vi "LightController.vi"() -> ()   [LabVIEW 2018]
uses:
  Content/TypeDef/EventTypeDef.ctl
  HASS-LV-WS_integration.lvlib
  <vilib>/MediaMongrels Ltd/WebSockets/WebSockets/WebSockets.lvlib
panel:
  in  "Pulse":bool
  out "Light State":T1
  in  "Color Temperature":u16(slide) scale=153.0..500.0
  in  "Brightness":u8(slide) scale=0.0..255.0
  in  "Light Entity ID":string
  in  "Light Control":bool
  out "Event Data":string
  out "Event Name":string
  in  "Stop Button":bool
  out "Connection Authenticated?":bool
  out "Connection Result":string
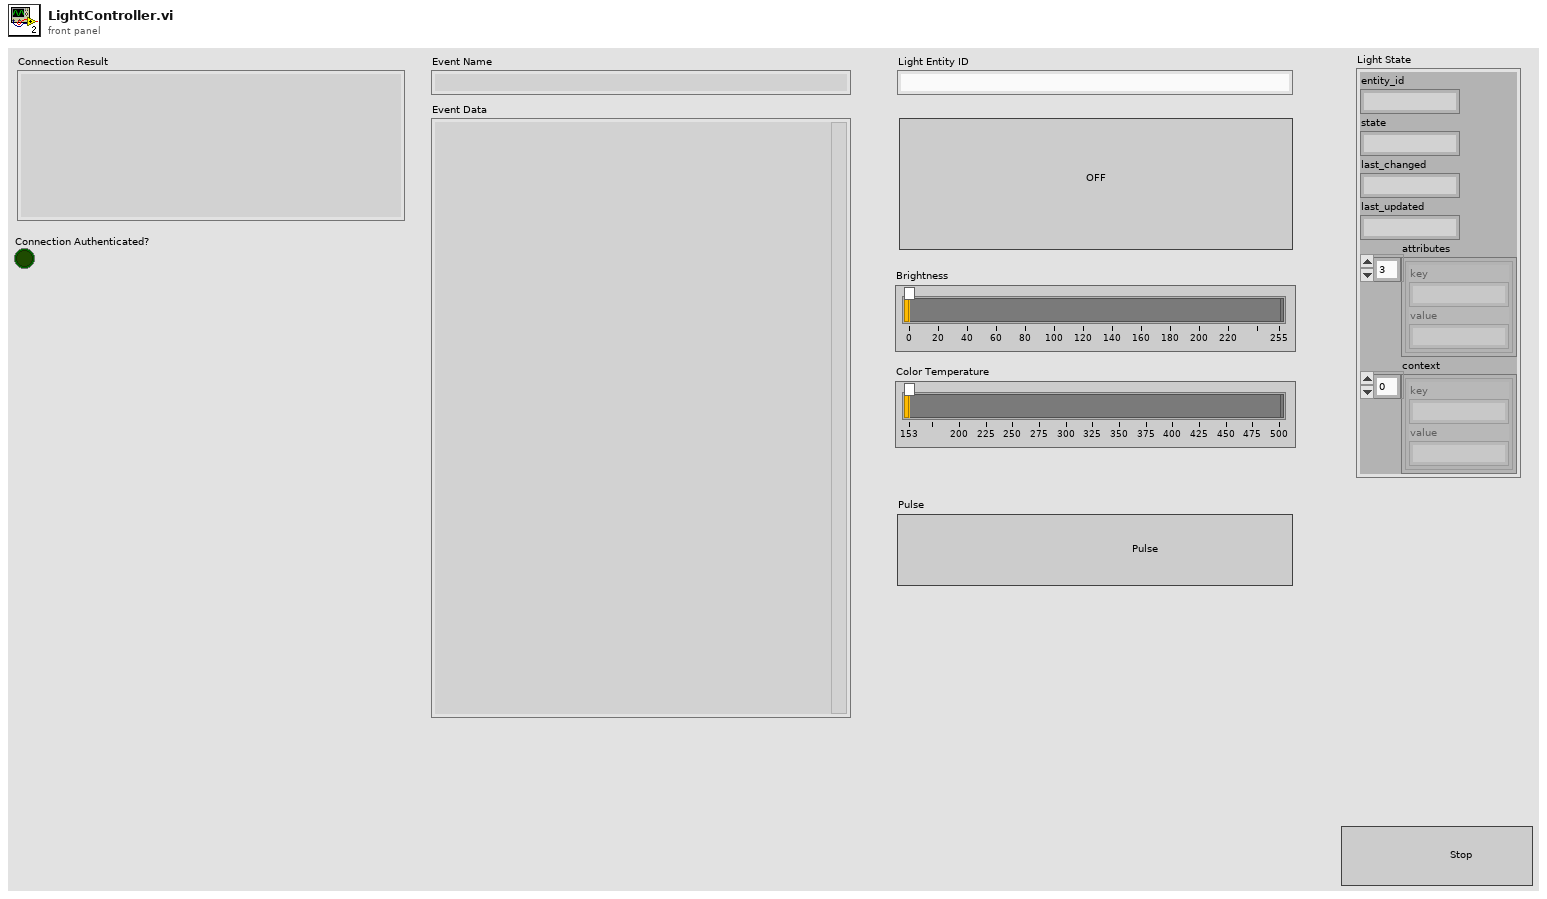
[diagram p1: front panel]
types:
  T1 = cluster{"entity_id":string, "state":string, "last_changed":string, "last_updated":string, "attributes":cluster{"key":string, "value":string}[], "context":cluster{"key":string, "value":string}[]}
  T2 = typedef "HASS-LV-WS_integration.lvlib/ReferencesTypeDef.ctl" = cluster{"user event":refnum<user-event>, "send queue":refnum<queue>, "receive queue":refnum<queue>, "TCP Network Connection":refnum<k5>, "ws engine notifier ":refnum<notifier>, "Event Registration Refnum":refnum<event-registration>}
  T3 = typedef "HASS-LV-WS_integration.lvlib/EventTypeDef.ctl" = cluster{"Data":variant, "Command":string}
  T4 = cluster{"Service Domain":string, "Service":string, "Optional - Service Data (JSON string)":string}
  T5 = cluster{"entity_id":string, "state":string, "last_changed":string, "last_updated":string, "attributes":cluster{"key":string, "value":string}[], "context":cluster{"key":string, "value":string}[]}[]
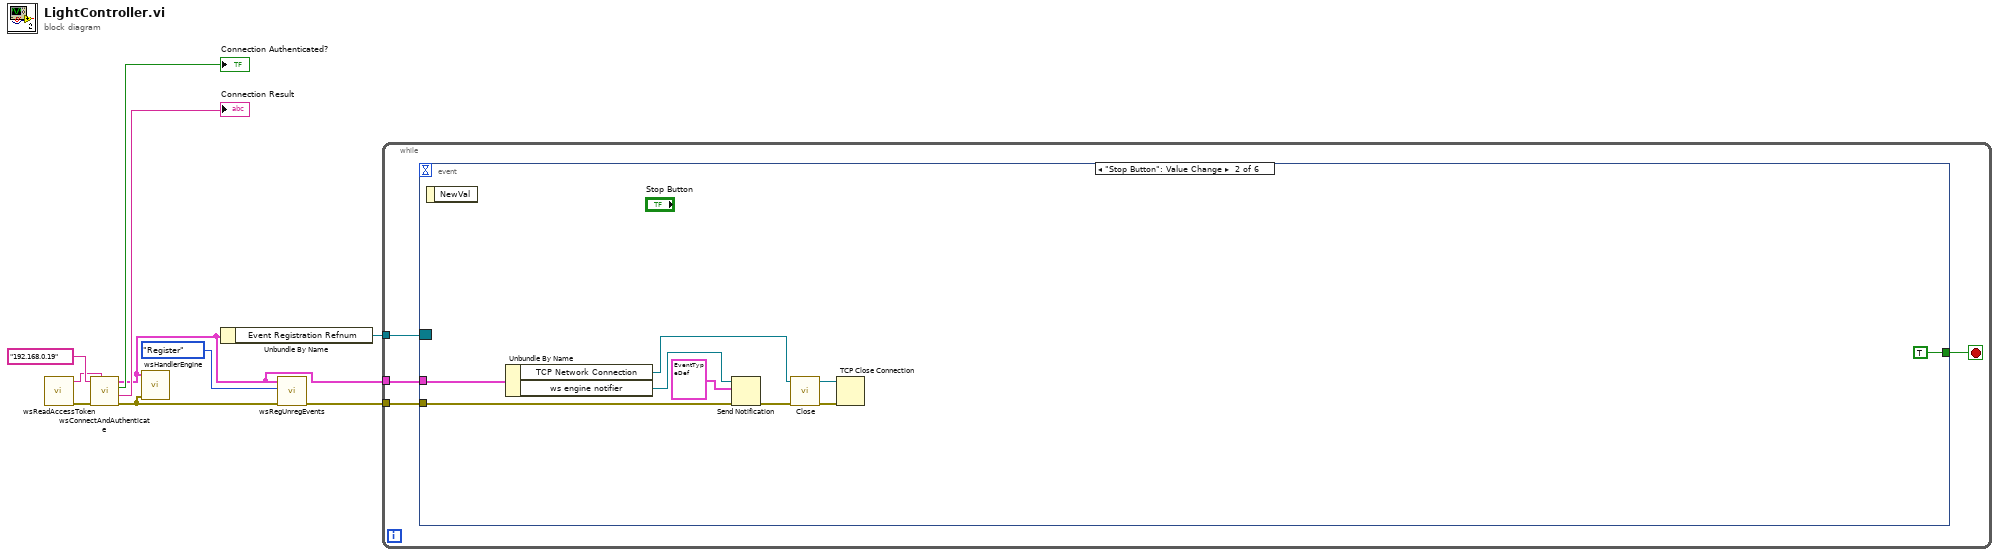
[diagram p0: block diagram]
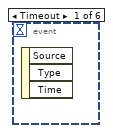
[diagram p2: hidden frame]
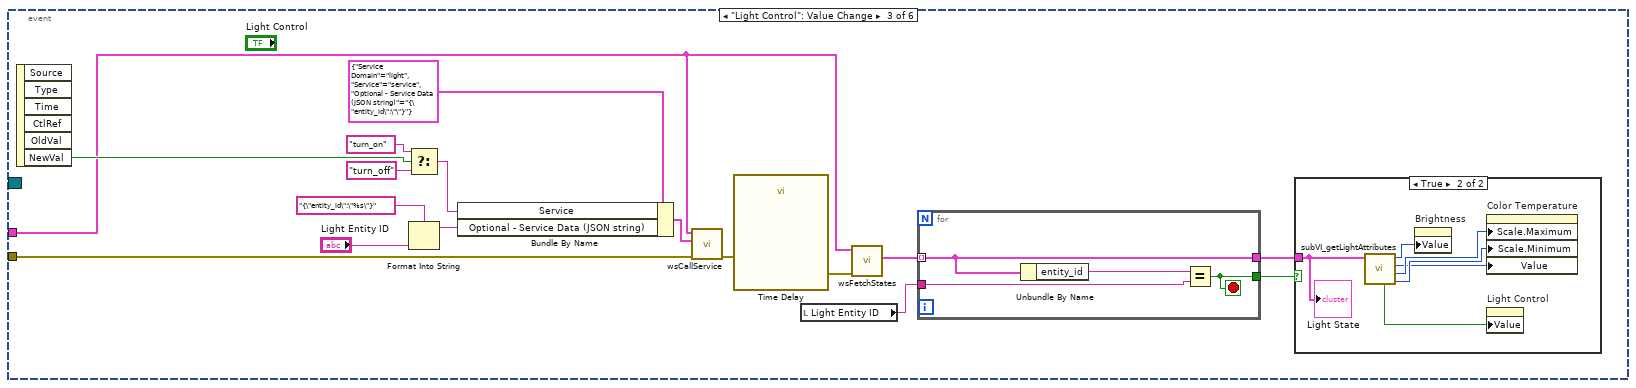
[diagram p3: hidden frame]
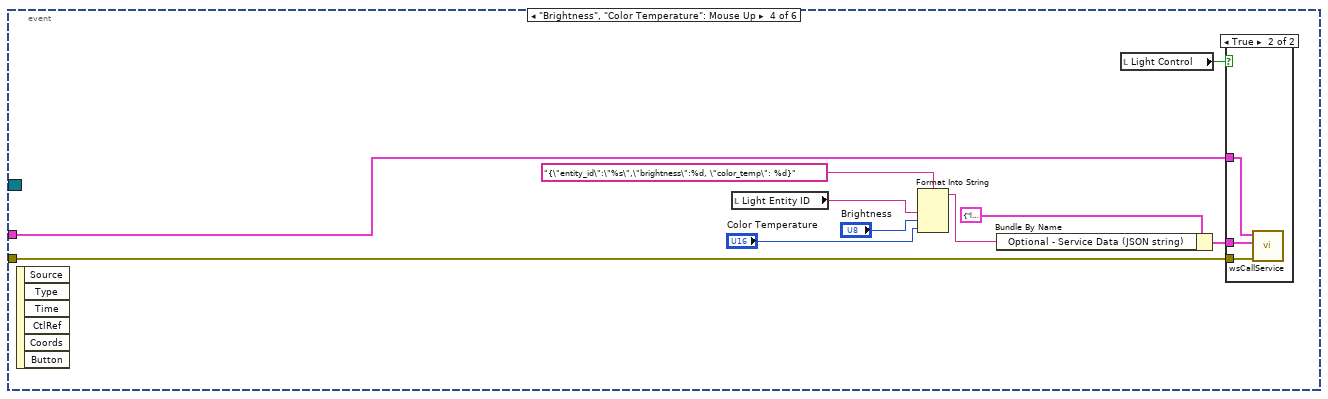
[diagram p5: hidden frame]
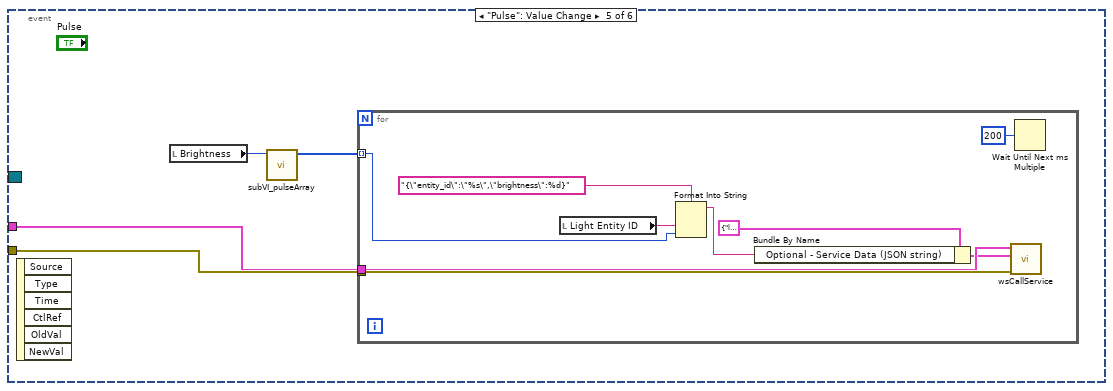
[diagram p7: hidden frame]
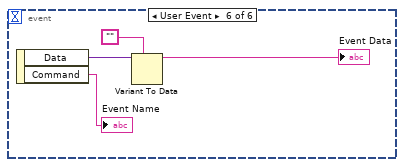
[diagram p8: hidden frame]
diagram:
  n1 = call "wsReadAccessToken.vi"() -> ("error out"=w6:errorcluster, "access token"=w5:string)  [unwired: 9 in, 1 out]
  n2 = call "wsConnectAndAuthenticate.vi"("Access Token"=w5, "error in (no error)"=w6, "Server Address"="192.168.0.19") -> ("error out"=w3:errorcluster, "Connection Result"=→"Connection Result":string, "Connection Authenticated?"=→"Connection Authenticated?":bool, "References"=w1:T2)  [unwired: 5 in]
  n3 = call "wsHandlerEngine.vi"("error in (no error)"=w3, "References"=w1) -> ()  [unwired: 9 in, 1 out]
  n4 = Unbundle By Name(w1) -> ("Event Registration Refnum"=w7:refnum<event-registration>)
  n5 = call "wsRegUnregEvents.vi"("Error In"=w3, "Action"=enum16{"Register", "Unregister"}."Register", "References"=w1) -> ("Error Out"=w2:errorcluster)  [unwired: 8 in]
  n6 = while {
    tunnel: w1 -> [w13]
    tunnel: w2 -> [w12]
    tunnel: w7 -> [w11]
    stop <- w14 stop-if-true
    n7 = event shown="[1] \"Stop Button\": Value Change" {
      selector: w11 -> [_ _ _ _ _ _]
      dyn-events: _ -> [_ _ _ _ _ _]
      timeout: _ -> [_ _ _ _ _ _]
      tunnel: [_ TRUE _ _ _ _] -> w14
      tunnel: w13 -> [_ w22 w26 w60 w66 _]
      tunnel: w12 -> [_ w20 w40 w59 w67 _]
      event Timeout {
        n8 = event-data() -> ()  [unwired: 1 in, 3 out]
      }
      event "Stop Button": Value Change {
        n9 = event-data() -> ()  [unwired: 1 in, 1 out]
        n10 = Unbundle By Name(w22) -> ("TCP Network Connection"=w17:refnum<k5>, "ws engine notifier"=w21:refnum<notifier>)
        n11 = Send Notification(notification=T3 {"Data"=variant, "Command"="Quit"}, notifier=w21, error in (no error)=w20) -> (error out=w19:errorcluster)  [unwired: 1 out]
        n12 = call <vilib>:"Close.vi"("error in (no error)"=w19, "WebSocket Connection in"=w17) -> ("error out"=w18:errorcluster, "WebSocket Connection in"=w16:refnum<k5>)  [unwired: 8 in]
        n13 = TCP Close Connection(connection ID=w16, error in (no error)=w18) -> ()  [unwired: 1 in, 2 out]
      }
      event "Light Control": Value Change {
        n14 = event-data() -> ("NewVal"=w37:bool)  [unwired: 1 in, 5 out]
        n15 = Select(t="turn_on" ("Service"), s=w37, f="turn_off") -> (s? t:f=w34:string)
        n16 = Format Into String(format string="{\"entity_id\":\"%s\"}" ("Optional - Service Data (JSON string)"), "Light Entity ID") -> (resulting string=w33:string)  [unwired: 2 in, 1 out]
        n17 = Bundle By Name(cluster=T4 {"Service Domain"="light", "Service"="service", "Optional - Service Data (JSON string)"="{\"entity_id\":\"\"}"} ("Call Service Data"), "Service"=w34, "Optional - Service Data (JSON string)"=w33) -> (w38:T4)
        n18 = call "wsCallService.vi"("error in (no error)"=w40, "Call Service Data"=w38, "References"=w26) -> ("error out"=w25:errorcluster)  [unwired: 7 in, 1 out]
        n19 = call "Time Delay"("error in (no error)"=w25) -> ("error out"=w24:errorcluster)  [unwired: 10 in]
        n20 = local read "Light Entity ID"() -> (w29:string)
        n21 = call "wsFetchStates.vi"("error in (no error)"=w24, "References"=w26) -> ("states"=w30:T5)  [unwired: 7 in, 2 out]
        n22 = for {
          tunnel: w30 -> [w47] mode=indexing
          tunnel: w29 -> [w49]
          tunnel: [w48] -> w27
          tunnel: [w47] -> w28
          stop <- w48 stop-if-true
          n23 = Unbundle By Name(w47) -> ("entity_id"=w50:string)
          n24 = Equal?(x=w50, y=w49) -> (x = y?=w48:bool)
        }
        n25 = case shown="True" w27 {
          tunnel: w28 -> [_ w46]
          frame False {
          }
          frame True {
            n26 = call "subVI_getLightAttributes.vi"("Cluster"=w46) -> ("min_mireds"=w42:i32, "max_mireds"=w43:i32, "color_temp"=w41:i32, "brightness"=w44:i32, "state"=w45:bool)  [unwired: 6 in]
            n27 = property on="Brightness" class="Slide (strict)"("Value"=w44) -> ()  [unwired: 2 in, 2 out]
            n28 = property on="Color Temperature" class="Slide (strict)"("Scale.Maximum"=w43, "Scale.Minimum"=w42, "Value"=w41) -> ()  [unwired: 2 in, 2 out]
            n29 = property on="Light Control" class="Bool (strict)"("Value"=w45) -> ()  [unwired: 2 in, 2 out]
            "Light State" <- w46
          }
        }
      }
      event "Brightness", "Color Temperature": Mouse Up {
        n30 = event-data() -> ()  [unwired: 1 in, 6 out]
        n31 = local read "Light Entity ID"() -> (w53:string)
        n32 = Format Into String(format string="{\"entity_id\":\"%s\",\"brightness\":%d, \"color_temp\": %d}", w53, "Brightness", "Color Temperature") -> (resulting string=w55:string)  [unwired: 2 in, 1 out]
        n33 = Bundle By Name(cluster=T4 {"Service Domain"="light", "Service"="turn_on", "Optional - Service Data (JSON string)"="{\"entity_id\":\"\"}"} ("Call Service Data"), "Optional - Service Data (JSON string)"=w55) -> (w57:T4)
        n34 = local read "Light Control"() -> (w51:bool)
        n35 = case shown="True" w51 {
          tunnel: w60 -> [_ w63]
          tunnel: w59 -> [_ w62]
          tunnel: w57 -> [_ w61]
          frame False {
          }
          frame True {
            n36 = call "wsCallService.vi"("error in (no error)"=w62, "Call Service Data"=w61, "References"=w63) -> ()  [unwired: 7 in, 2 out]
          }
        }
      }
      event "Pulse": Value Change {
        n37 = event-data() -> ()  [unwired: 1 in, 6 out]
        n38 = local read "Brightness"() -> (w65:u8)
        n39 = call "subVI_pulseArray.vi"("Brightness"=w65) -> ("Pulsearray"=w64:i32[])  [unwired: 10 in]
        n40 = for {
          tunnel: w67 -> [w72]
          tunnel: w66 -> [w71]
          tunnel: w64 -> [w69] mode=indexing
          n41 = local read "Light Entity ID"() -> (w75:string)
          n42 = Format Into String(format string="{\"entity_id\":\"%s\",\"brightness\":%d}", w75, w69) -> (resulting string=w76:string)  [unwired: 2 in, 1 out]
          n43 = Bundle By Name(cluster=T4 {"Service Domain"="light", "Service"="turn_on", "Optional - Service Data (JSON string)"="{\"entity_id\":\"\"}"} ("Call Service Data"), "Optional - Service Data (JSON string)"=w76) -> (w70:T4)
          n44 = call "wsCallService.vi"("error in (no error)"=w72, "Call Service Data"=w70, "References"=w71) -> ()  [unwired: 7 in, 2 out]
          n45 = Wait Until Next ms Multiple(millisecond multiple=u32 200) -> ()  [unwired: 1 out]
        }
      }
      event User Event {
        n46 = event-data() -> ("Data"=w79:variant, "Command"=→"Event Name":string)  [unwired: 1 in]
        n47 = Variant To Data(type="", Variant=w79) -> (data=→"Event Data":string)  [unwired: 1 in, 1 out]
      }
    }
  }
